vi "getWaveForm.vi"(0 "tiempo (s)":sgl, 1 "#samples":u32, 2 "Amplitud":dbl, 3 "frecuencia":dbl, 4 "Fs (S/s)":dbl, 5 "df":dbl[](array[numeric])) -> (6 "Inicial":dbl, 7 "Waveform":waveform(dbl), 8 "Ultimo":dbl)   [LabVIEW 2010]
panel:
  out "Numeric":i32
  out "#samples 2":u32
  out "size(s)":i32
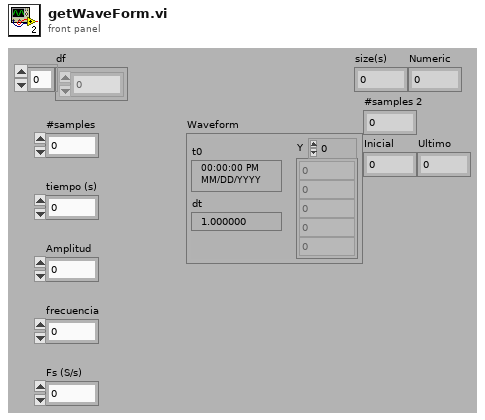
[diagram p1: front panel]
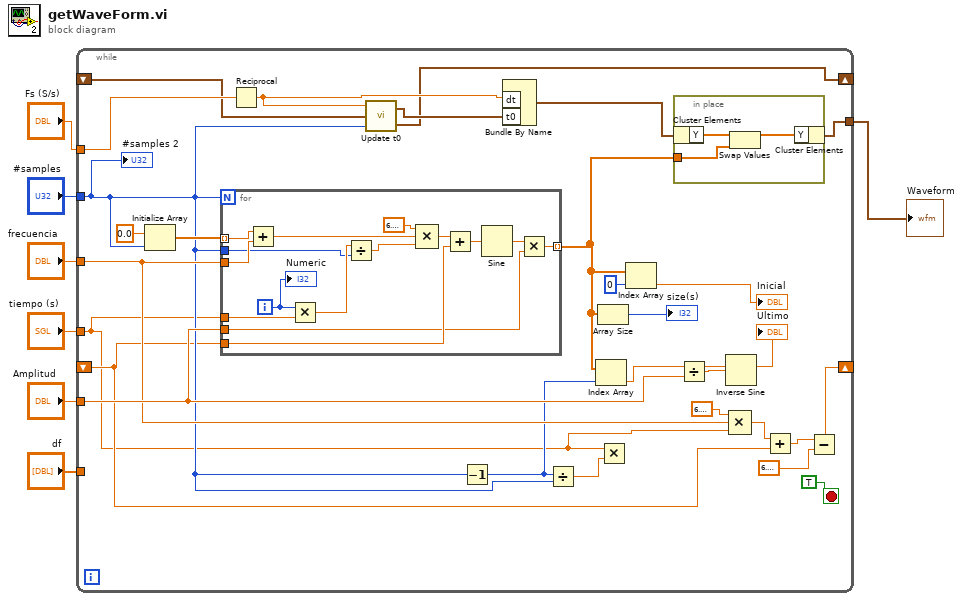
[diagram p0: block diagram]
diagram:
  n1 = while {
    tunnel: "#samples" -> [w18]
    tunnel: "tiempo (s)" -> [w8]
    tunnel: "frecuencia" -> [w32]
    tunnel: "Amplitud" -> [w34]
    shift-right: [w17] -> _
    shift-left: _ -> [w11]
    tunnel: "Fs (S/s)" -> [w29]
    shift-right: [w24] -> _
    shift-left: _ -> [w27]
    tunnel: [w23] -> w7
    tunnel: "df" -> [_]
    stop <- TRUE stop-if-true
    n2 = Initialize Array(0.0 ("element"), w18) -> (w20:dbl[])
    n3 = for {
      N: w18 -> [_]
      tunnel: w8 -> [w52]
      tunnel: w32 -> [w42]
      tunnel: [w47] -> w15 mode=indexing
      tunnel: w11 -> [w49]
      tunnel: w34 -> [w46]
      tunnel: w18 -> [w40]
      tunnel: w20 -> [w39] mode=indexing
      i -> [w53]
      n4 = Add(x=w39, y=w42) -> (x+y=w41:dbl)
      n5 = Multiply(x=w53, y=w52) -> (x*y=w51:sgl)
      n6 = Divide(x=w51, y=w40) -> (x/y=w44:sgl)
      n7 = Compound Arithmetic op=MULTIPLY(6.283185307179586, w41, w44) -> (w43:dbl)
      n8 = Add(x=w43, y=w49) -> (x+y=w50:dbl)
      n9 = Sine(x=w50) -> (sin(x)=w48:dbl)
      n10 = Multiply(x=w48, y=w46) -> (x*y=w47:dbl)
      "Numeric" <- w53
    }
    n11 = Reciprocal(x=w29) -> (1/x=w26:dbl)
    n12 = call "Update t0.vi"("#samples"=w18, "t0 IN"=w27, "dt"=w26) -> ("tf new"=w24:timestamp, "t0 OUT"=w25:timestamp)
    n13 = Decrement(x=w18) -> (x-1=w19:u32)
    n14 = Bundle By Name("dt"=w26, "t0"=w25) -> (w28:waveform(dbl))  [unwired: 1 in]
    n15 = Divide(x=w19, y=w18) -> (x/y=w16:dbl)
    n16 = Index Array(array=w15, index=w19) -> (element=w30:dbl)
    "Ultimo" <- w30
    n17 = Array Size(array=w15) -> (size(s)=→"size(s)":i32)
    n18 = Multiply(x=w8, y=w16) -> ()  [unwired: 1 out]
    n19 = Index Array(array=w15, index=0) -> (element=→"Inicial":dbl)
    n20 = in-place {
      in-place-border: w15 -> [w36]
      n21 = in-place-cluster #1(w28) -> ("Y"=w38:dbl[])
      n22 = Swap Values(12:w38, 14:w36) -> (1:w37:dbl[])  [unwired: 1 in, 1 out]
      n23 = in-place-cluster #1("Y"=w37) -> (w23:waveform(dbl))
    }
    n24 = Divide(x=w30, y=w34) -> (x/y=w31:dbl)
    n25 = Inverse Sine(1:w31) -> ()  [unwired: 1 out]
    n26 = Compound Arithmetic op=MULTIPLY(6.283185307179586, w32, w8) -> (w12:dbl)
    n27 = Add(x=w12, y=w11) -> (x+y=w9:dbl)
    n28 = Subtract(x=w9, y=6.283185307179586) -> (x-y=w17:dbl)
    "#samples 2" <- w18
  }
  "Waveform" <- w7
